vi "Append Link.vi"(8 "error in (no error)":errorcluster, 10 "Link":refnum<class "Link.lvclass">, 11 "Robot Arm in":refnum<class "Robot Arm.lvclass">) -> (0 "error out":errorcluster, 3 "Robot Arm out":refnum<class "Robot Arm.lvclass">)   [LabVIEW 2013, in "Robot Arm.lvclass"]
uses:
  Robot Arm.lvclass
  Link/Link.lvclass
  Robot Arm.lvclass/Robot Arm.ctl
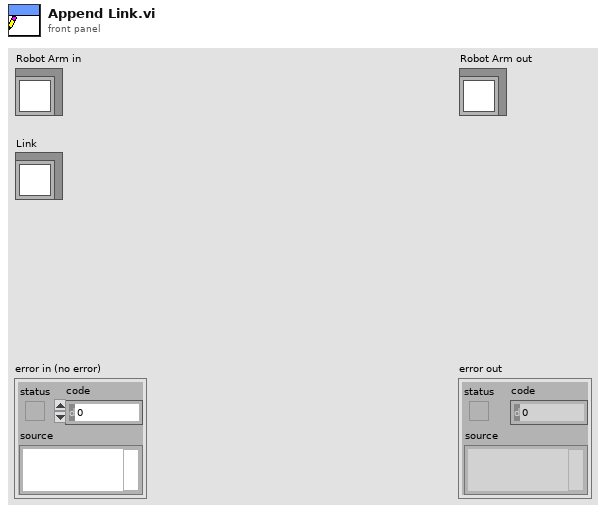
[diagram p1: front panel]
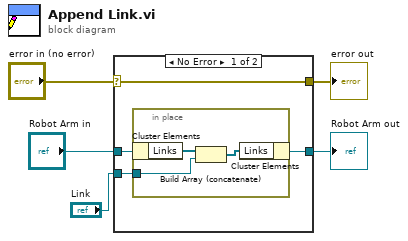
[diagram p0: block diagram]
diagram:
  n1 = case shown="No Error" "error in (no error)" {
    selector: "error in (no error)" -> [w9 w13]
    tunnel: [w9 w13] -> w4
    tunnel: [w7 w14] -> w2
    tunnel: "Robot Arm in" -> [w8 w14]
    tunnel: "Link" -> [w6 _]
    frame No Error {
      n2 = in-place {
        in-place-border: w6 -> [w12]
        n3 = in-place-cluster #1(w8) -> ("Links"=w11:refnum<class "Link.lvclass">[])
        n4 = Build Array (concatenate)(w11, w12) -> (w10:refnum<class "Link.lvclass">[])
        n5 = in-place-cluster #1("Links"=w10) -> (w7:refnum<class "Robot Arm.lvclass">)
      }
    }
    frame Error {
    }
  }
  "error out" <- w4
  "Robot Arm out" <- w2
